vi "Write and Read Serial Port(CH1603B).vi"(5 "Loop Read(3)":i32=3, 6 "Read Command Len(8)":i32=8, 7 "Delay Time(200ms)":u32=200, 8 "error in (no error)":errorcluster, 9 "Reply Flag Byte":u8=33 format="%02x", 10 "Write Command":string, 11 "VISA resource name in":refnum<visa-resource-name>) -> (0 "error out":errorcluster, 1 "Read String":string, 2 "Result(T:Pass)":bool, 3 "VISA resource name out":refnum<visa-resource-name>)   [LabVIEW 2015]
doc: "Write the command to serial port,then read the device replay command,check the result by read string length and reply flag byte."
panel:
  # "Write and Read Serial Port(CH1603B)"
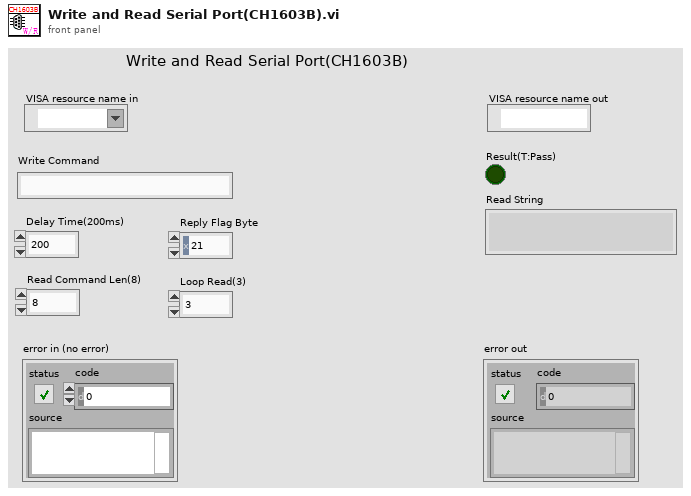
[diagram p1: front panel]
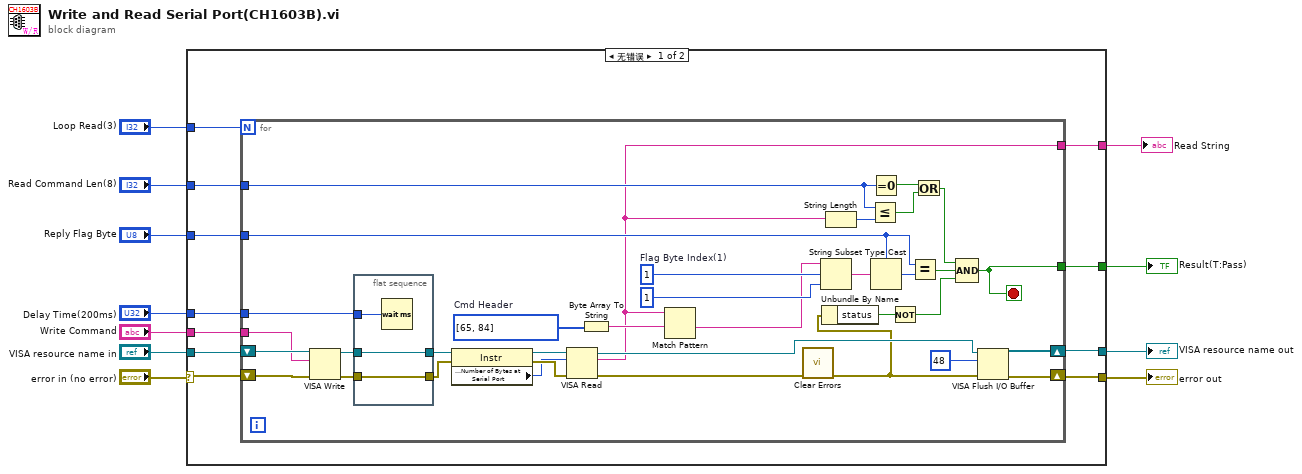
[diagram p0: block diagram]
diagram:
  n1 = case shown="无错误" "error in (no error)" {
    selector: "error in (no error)" -> [w22 w62]
    tunnel: "VISA resource name in" -> [w21 w61]
    tunnel: [w13 w62] -> w8
    tunnel: [w12 w61] -> w9
    tunnel: "Delay Time(200ms)" -> [w20 _]
    tunnel: [w19 _] -> w6
    tunnel: "Loop Read(3)" -> [w18 _]
    tunnel: [w17 _] -> w4
    tunnel: "Write Command" -> [w16 _]
    tunnel: "Reply Flag Byte" -> [w15 _]
    tunnel: "Read Command Len(8)" -> [w14 _]
    frame No Error {
      n2 = for {
        N: w18 -> [_]
        tunnel: w20 -> [w53]
        tunnel: [w27] -> w19
        shift-right: [w33] -> w13
        shift-left: w22 -> [w57]
        shift-right: [w32] -> w12
        shift-left: w21 -> [w56]
        tunnel: [w41] -> w17
        tunnel: w16 -> [w40]
        tunnel: w15 -> [w39]
        tunnel: w14 -> [w38]
        stop <- w41 stop-if-true
        w30 = u8[] [65, 84]  # Cmd Header
        w47 = 1  # Flag Byte Index(1)
        n3 = VISA Write(VISA resource name=w56, write buffer=w40, error in (no error)=w57) -> (VISA resource name out=w54:refnum<visa-resource-name>, error out=w55:errorcluster)  [unwired: 1 out]
        n4 = flat-sequence {
          tunnel: w55 -> [w59]
          tunnel: w54 -> [w58]
          tunnel: w53 -> [w60]
          tunnel: [w59] -> w52
          tunnel: [w58] -> w51
          frame #0 {
            n5 = Wait (ms)(milliseconds to wait=w60) -> ()  [unwired: 1 out]
          }
        }
        n6 = property on="Property Node" class="Instr"(reference=w51, error in=w52) -> (reference out=w49:refnum<visa-resource-name>, error out=w50:errorcluster, "Serial Settings:Number of Bytes at Serial Port"=w48:u32)
        n7 = VISA Read(VISA resource name=w49, byte count=w48, error in (no error)=w50) -> (VISA resource name out=w31:refnum<visa-resource-name>, read buffer=w27:string, error out=w26:errorcluster)  [unwired: 1 out]
        n8 = Byte Array To String(unsigned byte array=w30) -> (string=w29:string)
        n9 = Match Pattern(string=w27, regular expression=w29) -> (after substring=w28:string)  [unwired: 1 in, 3 out]
        n10 = call <vilib>:"Clear Errors.vi"("error in (no error)"=w26) -> ("error out"=w23:errorcluster)  [unwired: 5 in, 1 out]
        n11 = String Subset(string=w28, offset (0)=w47, length (rest)=1 ("长度（剩余）")) -> (substring=w45:string)
        n12 = Unbundle By Name(w23) -> ("status"=w25:bool)
        n13 = String Length(string=w27) -> (length=w43:i32)
        n14 = Less Or Equal?(x=w38, y=w43) -> (x <= y?=w36:bool)
        n15 = Equal To 0?(x=w38) -> (x = 0?=w37:bool)
        n16 = Type Cast(type=w39, x=w45) -> (*(type *) &x=w44:u8)
        n17 = Not(x=w25) -> (.not. x?=w24:bool)
        n18 = Equal?(x=w39, y=w44) -> (x = y?=w42:bool)
        n19 = Or(x=w37, y=w36) -> (x .or. y?=w35:bool)
        n20 = Compound Arithmetic op=AND ("复合运算")(w35, w42, w24) -> (w41:bool)
        n21 = VISA Flush I/O Buffer(VISA resource name=w31, mask (16)=u16 48 ("长度（剩余）"), error in (no error)=w23) -> (VISA resource name out=w32:refnum<visa-resource-name>, error out=w33:errorcluster)
      }
    }
    frame Error {
    }
  }
  "VISA resource name out" <- w9
  "error out" <- w8
  "Read String" <- w6
  "Result(T:Pass)" <- w4
